vi "Range Minimum Write.vi"(6 "Control Ref Queue":T1, 8 "error in (no error)":errorcluster, 9 "Range Min":sgl, 11 "3D Plot.lvclass in":refnum<class "3D Plot.lvclass">) -> (0 "error out":errorcluster, 3 "3D Plot.lvclass out":refnum<class "3D Plot.lvclass">)   [LabVIEW 2020, in "3D Plot.lvclass"]
uses:
  3D Plot.lvclass
  3DMathPlot Ctrl Act Queue.ctl
  3DMathPlot Ctrl Act Cluster.ctl
  3DMathPlot State Class.ctl
  3D Plot.lvclass/3D Plot.ctl
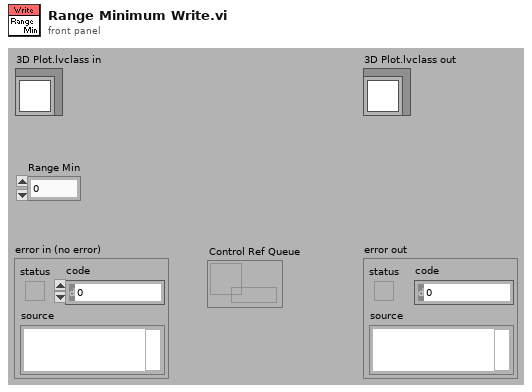
[diagram p1: front panel]
types:
  T1 = typedef "3DMathPlot Ctrl Act Queue.ctl" = refnum<queue>
  T2 = typedef "3D Plot.lvclass/Range Clusters.ctl" = cluster{"X Range":cluster{"Max X":sgl, "Min X":sgl}, "Y Range":cluster{"Max Y":sgl, "Min Y":sgl}, "Z Range":cluster{"Max Z":sgl, "Min Z":sgl}}
  T3 = cluster{"Auto Range X":bool, "Auto Range Y":bool, "Auto Range Z":bool}
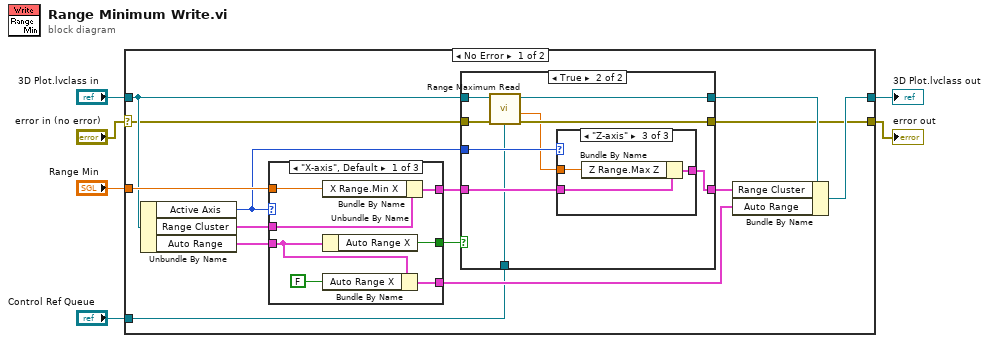
[diagram p0: block diagram]
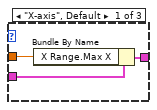
[diagram p3: hidden frame]
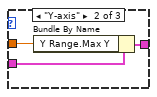
[diagram p4: hidden frame]
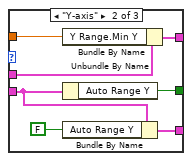
[diagram p5: hidden frame]
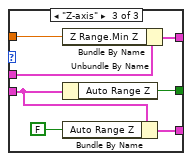
[diagram p6: hidden frame]
diagram:
  n1 = case shown="No Error" "error in (no error)" {
    selector: "error in (no error)" -> [w13 w63]
    tunnel: "Range Min" -> [w20 _]
    tunnel: "3D Plot.lvclass in" -> [w15 w64]
    tunnel: [w18 w64] -> w4
    tunnel: [w12 w63] -> w2
    tunnel: "Control Ref Queue" -> [w11 _]
    frame No Error {
      n2 = Unbundle By Name(w15) -> ("Active Axis"=w10:enum16{"X-axis", "Y-axis", "Z-axis"}, "Range Cluster"=w19:T2, "Auto Range"=w17:T3)
      n3 = case shown="\"X-axis\", Default" w10 {
        tunnel: w19 -> [w48 w53 w61]
        tunnel: w20 -> [w47 w55 w62]
        tunnel: [w46 w54 w60] -> w9
        tunnel: w17 -> [w44 w51 w58]
        tunnel: [w43 w49 w57] -> w7
        tunnel: [w42 w50 w56] -> w16
        frame "X-axis", Default {
          n4 = Bundle By Name(cluster=w48, "X Range.Min X"=w47) -> (w46:T2)
          n5 = Unbundle By Name(w44) -> ("Auto Range X"=w43:bool)
          n6 = Bundle By Name(cluster=w44, "Auto Range X"=FALSE) -> (w42:T3)
        }
        frame "Y-axis" {
          n7 = Bundle By Name(cluster=w53, "Y Range.Min Y"=w55) -> (w54:T2)
          n8 = Unbundle By Name(w51) -> ("Auto Range Y"=w49:bool)
          n9 = Bundle By Name(cluster=w51, "Auto Range Y"=FALSE ("Auto Range X")) -> (w50:T3)
        }
        frame "Z-axis" {
          n10 = Bundle By Name(cluster=w61, "Z Range.Min Z"=w62) -> (w60:T2)
          n11 = Unbundle By Name(w58) -> ("Auto Range Z"=w57:bool)
          n12 = Bundle By Name(cluster=w58, "Auto Range Z"=FALSE ("Auto Range X")) -> (w56:T3)
        }
      }
      n13 = case shown="True" w7 {
        tunnel: w15 -> [w23 w29]
        tunnel: [w23 w27] -> w14
        tunnel: w13 -> [w22 w28]
        tunnel: [w22 w26] -> w12
        tunnel: w10 -> [_ w32]
        tunnel: w9 -> [w21 w31]
        tunnel: [w21 w30] -> w8
        tunnel: w11 -> [_ w25]
        frame False {
        }
        frame True {
          n14 = call "Range Maximum Read.vi"("Control Ref Queue"=w25, "error in (no error)"=w28, "3D Plot.lvclass in"=w29) -> ("error out"=w26:errorcluster, "Range Max"=w24:sgl, "3D Plot.lvclass out"=w27:refnum<class "3D Plot.lvclass">)  [unwired: 6 out]
          n15 = case shown="\"Z-axis\"" w32 {
            tunnel: w31 -> [w35 w38 w41]
            tunnel: [w33 w37 w39] -> w30
            tunnel: w24 -> [w34 w36 w40]
            frame "X-axis", Default {
              n16 = Bundle By Name(cluster=w35, "X Range.Max X"=w34) -> (w33:T2)
            }
            frame "Y-axis" {
              n17 = Bundle By Name(cluster=w38, "Y Range.Max Y"=w36) -> (w37:T2)
            }
            frame "Z-axis" {
              n18 = Bundle By Name(cluster=w41, "Z Range.Max Z"=w40) -> (w39:T2)
            }
          }
        }
      }
      n19 = Bundle By Name(cluster=w14, "Range Cluster"=w8, "Auto Range"=w16) -> (w18:refnum<class "3D Plot.lvclass">)
    }
    frame Error {
    }
  }
  "error out" <- w2
  "3D Plot.lvclass out" <- w4
